vi "NewGetRobotMode.vi"() -> (2 "Auton":bool, 3 "Disabled":bool)   [LabVIEW 2014]
doc: "This VI waits for control packets to arrive and determines what robot code to execute next, teletop, disable, etc. It also contains a state machine to give a first and last call context parameter and execution timings to robot code.\n\nThis software is licensed. Open the labview\\readme\\WPI Robotics Library Open Source License.txt file for more information."
panel:
  # "Andrew wrote this VI"
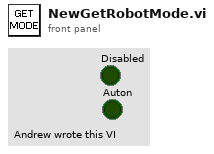
[diagram p1: front panel]
types:
  T1 = typedef "NetComm_ControlWord.ctl" = cluster{"Enabled":bool, "Autonomous":bool, "Test":bool, "E-Stop":bool, "FMS Attached":bool, "DS Attached":bool}
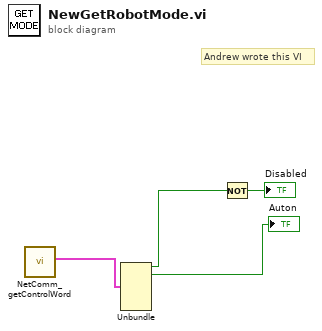
[diagram p0: block diagram]
diagram:
  # "Andrew wrote this VI"
  n1 = call <vilib>:"NetComm_getControlWord.vi"() -> ("Control Word"=w4:T1)  [unwired: 10 in, 1 out]
  n2 = Unbundle(w4) -> ("Enabled"=w3:bool, "Autonomous"=→"Auton":bool)  [unwired: 4 out]
  n3 = Not(x=w3) -> (.not. x?=→"Disabled":bool)
